vi "pH get titration values.vi"() -> (0 "canceled":bool=TRUE, 1 "Titration":T1 {"Nt" format="%.4f"; "Vo" format="%.3f"})   [LabVIEW 2015]
uses:
  pH titration.ctl
  pH gran type.ctl
panel:
  in  "Titration settings":T1 {"Nt" format="%.4f"; "Vo" format="%.3f"}
  out "Suggested Delta Va":dbl=nan format="%.3f"
  in  "cancel":bool
  in  "done":bool
  # "Maximum incremental volume of acid for 3 good points"
  # "mL"
  # "Normality of titrant"
  # "eq/L"
  # "mL"
  # "Volume of sample"
  # "Normality of titrant"
  # "eq/L"
  # "mL"
  # "Volume of sample"
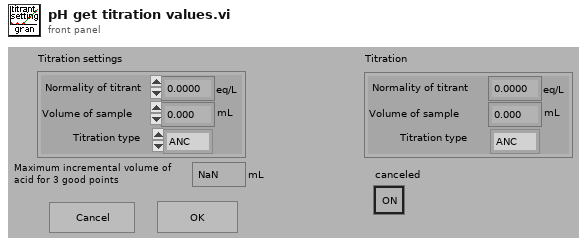
[diagram p1: front panel]
types:
  T1 = typedef "pH titration.ctl" = cluster{"Vo":dbl, "Nt":dbl, "Titration type":T2}
  T2 = typedef "pH gran type.ctl" = enum16{"ANC", "BNC"}
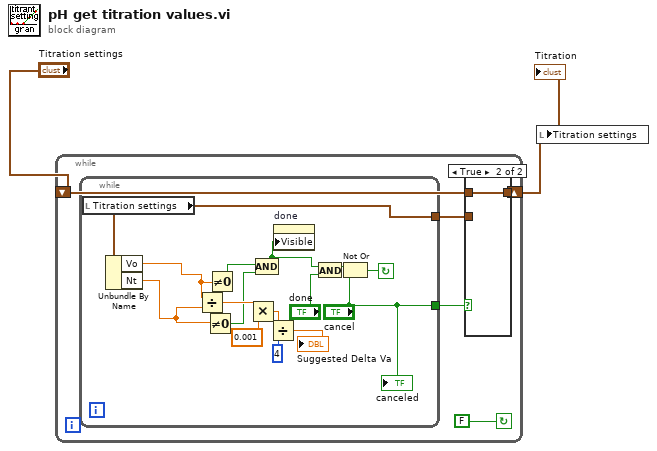
[diagram p0: block diagram]
diagram:
  n1 = while {
    shift-left: "Titration settings" -> [w6]
    shift-right: [w5] -> w1
    stop <- FALSE continue-if-true
    n2 = while {
      tunnel: [w8] -> w4
      tunnel: ["cancel"] -> w7
      stop <- w9 continue-if-true
      n3 = local read "Titration settings"() -> (w8:T1)
      n4 = Unbundle By Name(w8) -> ("Vo"=w14:dbl, "Nt"=w13:dbl)
      n5 = Divide(x=w14, y=w13) -> (x/y=w18:dbl)
      n6 = Not Equal To 0?(x=w13) -> (x != 0?=w12:bool)
      n7 = Not Equal To 0?(x=w14) -> (x != 0?=w11:bool)
      n8 = Multiply(x=w18, y=0.001) -> (x*y=w21:dbl)
      n9 = Compound Arithmetic op=AND(w11, w12) -> (w10:bool)
      n10 = Divide(x=w21, y=4) -> (x/y=→"Suggested Delta Va":dbl)
      n11 = property on="done" class="Bool"("Visible"=w10) -> ()  [unwired: 2 in, 2 out]
      n12 = And(x=w10, y="done") -> (x .and. y?=w22:bool)
      n13 = Not Or(1:"cancel", 2:w22) -> (0:w9:bool)
      "canceled" <- "cancel"
    }
    n14 = case shown="True" w7 {
      tunnel: w6 -> [_ w24]
      tunnel: [w23 w24] -> w5
      tunnel: w4 -> [w23 _]
      frame False {
      }
      frame True {
      }
    }
  }
  "Titration" <- w1
  n15 = local write "Titration settings"(w1) -> ()
